vi "SaveLog.vi"(8 "错误输入（无错误）":errorcluster, 11 "AllControls In":T1) -> (0 "错误输出":errorcluster)   [LabVIEW 2017]
uses:
  Ctrls/AllControls.ctl
  Ctrls/PathChoose.ctl
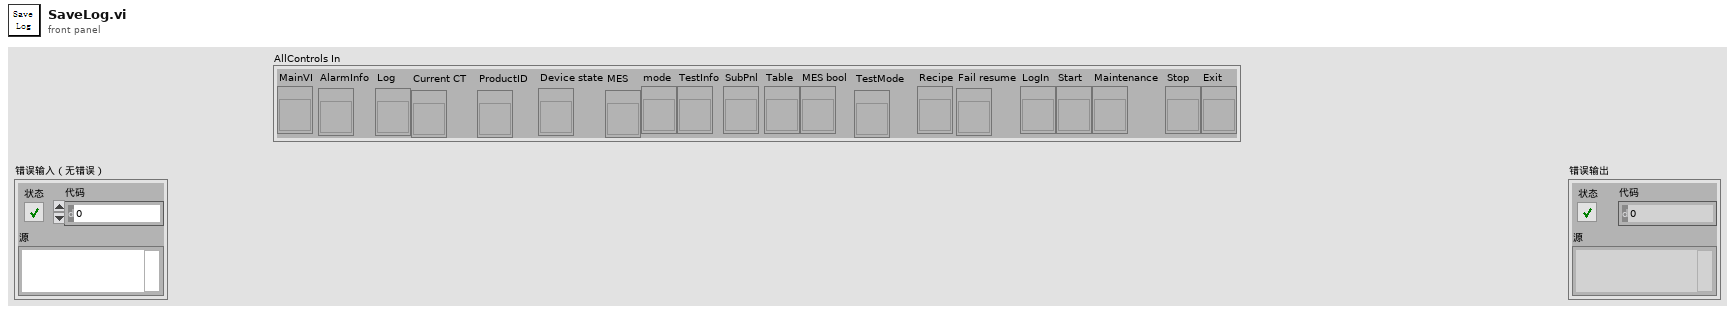
[diagram p1: front panel]
types:
  T1 = typedef "AllControls.ctl" = cluster{"MainVI":refnum<vi>, "AlarmInfo":refnum<vi>, "Log":refnum<vi>, "Current CT":refnum<vi>, "ProductID":refnum<vi>, "Device state":refnum<vi>, "MES":refnum<vi>, "mode":refnum<vi>, "TestInfo":refnum<vi>, "SubPnl":refnum<vi>, "Table":refnum<vi>, "MES bool":refnum<vi>, "TestMode":refnum<vi>, "Recipe":refnum<vi>, "Fail resume":refnum<vi>, "LogIn":refnum<vi>, "Start":refnum<vi>, "Maintenance":refnum<vi>, "Stop":refnum<vi>, "Exit":refnum<vi>}
  T2 = typedef "amc_Message Queue.ctl" = refnum<queue>
  T3 = typedef "PathChoose.ctl" = enum16{"OperatorLog", "AutoRunLog", "AlmLog", "TestData", "AllTestData", "backup_nvm", "backup_before_flashing"}
  T4 = enum16{"open", "replace", "create", "open or create", "replace or create", "replace or create with confirmation"}
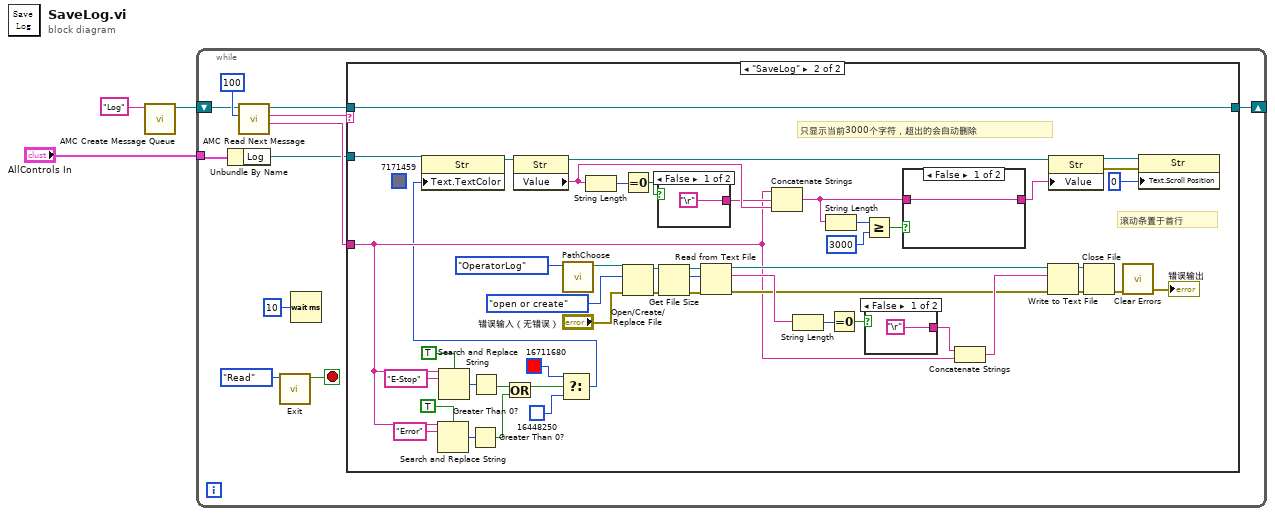
[diagram p0: block diagram]
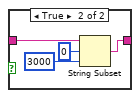
[diagram p3: hidden frame]
diagram:
  n1 = call "AMC Create Message Queue.vi"("Message Queue Name"="Log" ("Message queue name (unnamed)")) -> ("Message Queue out"=w3:T2)  [unwired: 4 in, 6 out]
  n2 = while {
    shift-right: [w10] -> _
    shift-left: w3 -> [w12]
    tunnel: "AllControls In" -> [w8]
    stop <- w5 stop-if-true
    n3 = Unbundle By Name(w8) -> ("Log"=w6:refnum<vi>)
    n4 = call "AMC Read Next Message.vi"("timeout (1ms)"=100 ("Timeout"), "Message Queue in"=w12) -> ("Message Value"=w7:string, "Message Name"=w11:string, "Message Queue out"=w9:T2)  [unwired: 2 in, 5 out]
    n5 = call "Exit.vi"("Step"=enum16{"Initial", "Write", "Read"}."Read" ("step")) -> ("Exit Out"=w5:bool)  [unwired: 9 in, 1 out]
    n6 = Wait (ms)(milliseconds to wait=u32 10) -> ()  [unwired: 1 out]
    n7 = case shown="\"SaveLog\"" w11 {
      tunnel: [w15 w64] -> w10
      tunnel: w9 -> [w15 w64]
      tunnel: w7 -> [_ w17]
      tunnel: w6 -> [_ w29]
      frame "假", Default {
      }
      frame "SaveLog" {
        (unwired) u32 7171459 ("TextColor")
        # "只显示当前3000个字符，超出的会自动删除"
        # "滚动条置于首行"
        n8 = Search and Replace String(case sensitive?=TRUE ("忽略大小写？(F)"), input string=w17, search string="Error") -> (number of replacements=w26:i32)  [unwired: 5 in, 3 out]
        n9 = Search and Replace String(case sensitive?=TRUE ("忽略大小写？(F)"), input string=w17, search string="E-Stop") -> (number of replacements=w24:i32)  [unwired: 5 in, 3 out]
        n10 = Greater Than 0?(x=w26) -> (x > 0?=w28:bool)
        n11 = Greater Than 0?(x=w24) -> (x > 0?=w25:bool)
        n12 = Or(x=w25, y=w28) -> (x .or. y?=w27:bool)
        n13 = Select(t=u32 16711680 ("TextColor"), s=w27, f=u32 16448250 ("TextColor")) -> (s? t:f=w16:u32)
        n14 = property class="Str"(reference=w29, "Text.TextColor"=w16) -> (reference out=w62:refnum<vi>)  [unwired: 1 in, 1 out]
        n15 = property class="Str"(reference=w62) -> (reference out=w35:refnum<vi>, "Value"=w53:string)  [unwired: 1 in, 1 out]
        n16 = call "PathChoose.vi"(11:PathChoose."OperatorLog") -> ("Path_Out"=w52:path)  [unwired: 10 in]
        n17 = String Length(string=w53) -> (length=w34:i32)
        n18 = Equal To 0?(x=w34) -> (x = 0?=w36:bool)
        n19 = Open/Create/Replace File(file path (use dialog)=w52, error in="错误输入（无错误）", operation (0:open)=T4."open or create" ("操作(0:open)")) -> (refnum out=w38:refnum<file>, error out=w39:errorcluster)  [unwired: 3 in, 1 out]
        n20 = case shown="False" w36 {
          tunnel: ["\r" _] -> w37
          frame False {
          }
          frame True {
          }
        }
        n21 = Get File Size ("获取文件大小")(file=w38, error in=w39) -> (refnum out=w40:refnum<file>, size (in bytes)=w42:i64, 0:w41:errorcluster)
        n22 = Read from Text File ("读取文本文件")(file (use dialog)=w40, count=w42, error in=w41) -> (refnum out=w43:refnum<file>, text=w47:string, error out=w44:errorcluster)  [unwired: 1 in, 1 out]
        n23 = Concatenate Strings(w17, w37, w53) -> (w58:string)
        n24 = String Length(string=w47) -> (length=w46:i32)
        n25 = String Length(string=w58) -> (length=w56:i32)
        n26 = Equal To 0?(x=w46) -> (x = 0?=w45:bool)
        n27 = Greater Or Equal?(x=w56, y=3000) -> (x >= y?=w57:bool)
        n28 = case shown="False" w45 {
          tunnel: ["\r" _] -> w48
          frame False {
          }
          frame True {
          }
        }
        n29 = case shown="False" w57 {
          tunnel: w58 -> [w65 w69]
          tunnel: [w65 w66] -> w59
          frame False {
          }
          frame True {
            n30 = String Subset(string=w69, offset (0)=0 ("偏移量(0)"), length (rest)=3000 ("长度（剩余）")) -> (substring=w66:string)
          }
        }
        n31 = Concatenate Strings(w48, w17) -> (w49:string)
        n32 = Write to Text File ("写入文本文件")(file (use dialog)=w43, text=w49, error in=w44) -> (refnum out=w50:refnum<file>, error out=w51:errorcluster)  [unwired: 1 in, 1 out]
        n33 = property class="Str"(reference=w35, "Value"=w59) -> (reference out=w60:refnum<vi>, error out=w61:errorcluster)  [unwired: 1 in]
        n34 = Close File(refnum=w50, error in=w51) -> (error out=w55:errorcluster)  [unwired: 1 out]
        n35 = call <vilib>:"Clear Errors.vi"("error in (no error)"=w55) -> ("error out"=→"错误输出":errorcluster)  [unwired: 5 in, 1 out]
        n36 = property class="Str"(reference=w60, error in=w61, "Text.Scroll Position"=u32 0 ("文本.滚动条位置")) -> ()  [unwired: 2 out]
      }
    }
  }
